vi "SetScaleAndOriginToCenterImage.vi"(0 "reference in":refnum<class "LcPictureBox.lvclass">, 2 "ImageFile":path, 3 "Image":refnum<k24>, 5 "Error In":errorcluster, 8 "UpdateScaleAndOrigin(True)":bool=TRUE) -> (14 "reference out":refnum<class "LcPictureBox.lvclass">, 15 "ScaleFactorUsed":sgl=1.0, 17 "OriginUsed":cluster{"x":sgl, "y":sgl}, 19 "Error Out":errorcluster)   [LabVIEW 2020, in "LcPictureBox.lvclass"]
uses:
  LcPictureBox.lvclass
  System.Drawing
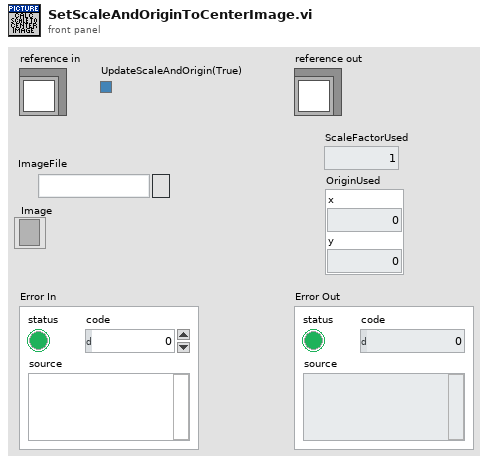
[diagram p1: front panel]
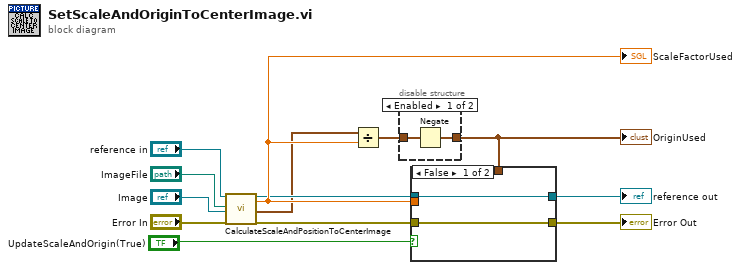
[diagram p0: block diagram]
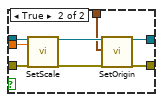
[diagram p3: hidden frame]
diagram:
  n1 = call-dynamic "CalculateScaleAndPositionToCenterImage.vi"("reference in"="reference in", "ImageFile"="ImageFile", "Image"="Image", "Error In"="Error In") -> ("reference out"=w3:refnum<class "LcPictureBox.lvclass">, "ScaleFactor"=w8:sgl, "ImagePosition"=w1:cluster{"x":sgl, "y":sgl}, "Error Out"=w2:errorcluster)  [unwired: 12 in]
  "ScaleFactorUsed" <- w8
  n2 = Divide(x=w1, y=w8) -> (x/y=w4:cluster{"x":sgl, "y":sgl})
  n3 = disable-structure shown="Enabled" {
    disable-tunnel: [w15 w16] -> w7
    disable-tunnel: w4 -> [w14 w16]
    frame Enabled {
      n4 = Negate(x=w14) -> (-x=w15:cluster{"x":sgl, "y":sgl})
    }
    frame Disabled {
    }
  }
  "OriginUsed" <- w7
  n5 = case shown="False" "UpdateScaleAndOrigin(True)" {
    tunnel: w3 -> [w17 w24]
    tunnel: w2 -> [w18 w23]
    tunnel: w8 -> [_ w22]
    tunnel: w7 -> [_ w21]
    tunnel: [w17 w20] -> w11
    tunnel: [w18 w19] -> w13
    frame False {
    }
    frame True {
      n6 = call-dynamic "SetScale.vi"("reference in"=w24, "ScaleFactor"=w22, "Error In"=w23) -> ("reference out"=w25:refnum<class "LcPictureBox.lvclass">, "Error Out"=w26:errorcluster)  [unwired: 15 in]
      n7 = call-dynamic "SetOrigin.vi"("reference in"=w25, "Origin"=w21, "Error In"=w26) -> ("reference out"=w20:refnum<class "LcPictureBox.lvclass">, "Error Out"=w19:errorcluster)  [unwired: 15 in]
    }
  }
  "Error Out" <- w13
  "reference out" <- w11
